vi "ge_Val2String_1Chan.vi"(0 "Value":u16, 1 "ColType":T1) -> (5 "String and Val":cluster{"String":string, "Value":u16})   [LabVIEW 2012]
uses:
  Custom Ctls Table/ge_ColType.ctl
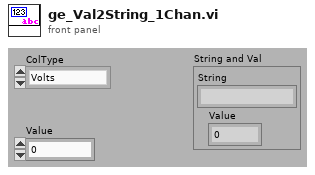
[diagram p1: front panel]
types:
  T1 = typedef "ge_ColType.ctl" = enum16{"Volts", "Amps", "Ohms", "TermCfg", "WireCfg", "Coup", "Slope", "Iex", "CalUnits", "ThrmUnits", "ThrmType", "CJCSrc", "BrdgType", "Strn Mode", "RTDType"}
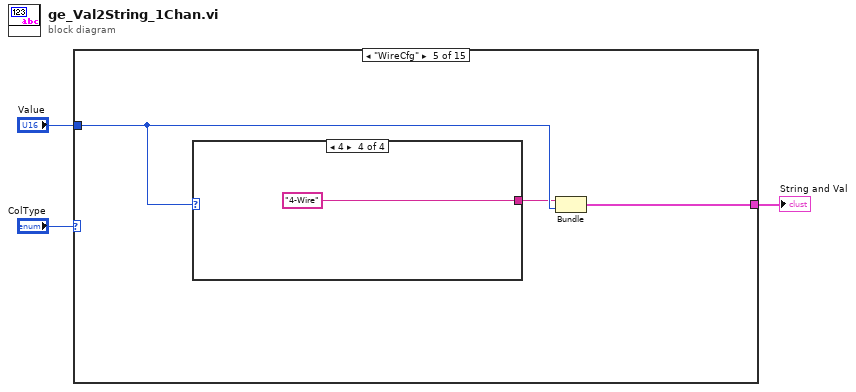
[diagram p0: block diagram]
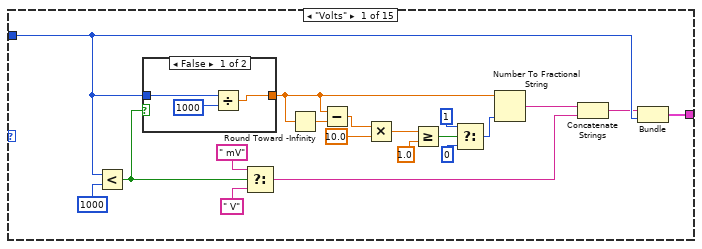
[diagram p2: hidden frame]
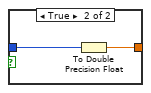
[diagram p3: hidden frame]
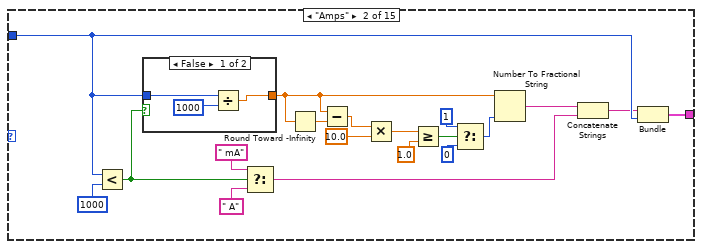
[diagram p4: hidden frame]
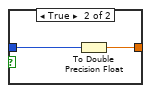
[diagram p5: hidden frame]
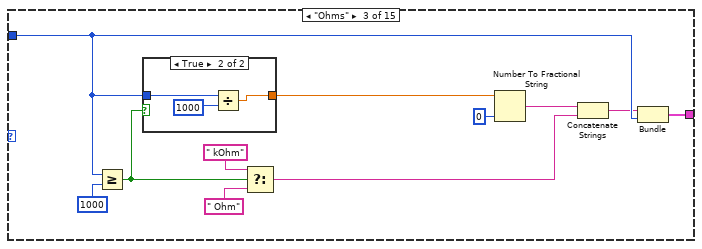
[diagram p6: hidden frame]
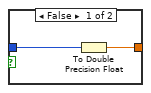
[diagram p7: hidden frame]
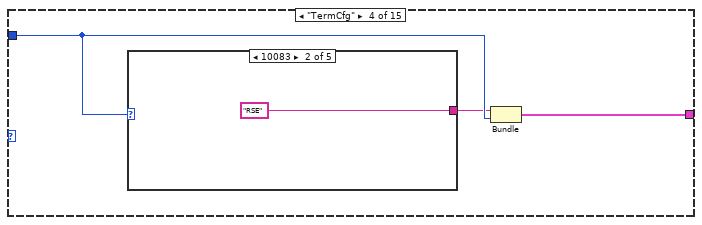
[diagram p8: hidden frame]
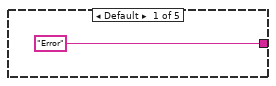
[diagram p9: hidden frame]
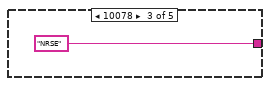
[diagram p10: hidden frame]
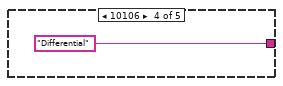
[diagram p11: hidden frame]
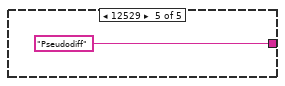
[diagram p12: hidden frame]
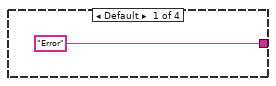
[diagram p13: hidden frame]
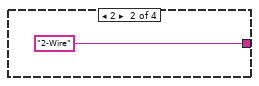
[diagram p14: hidden frame]
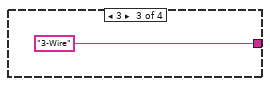
[diagram p15: hidden frame]
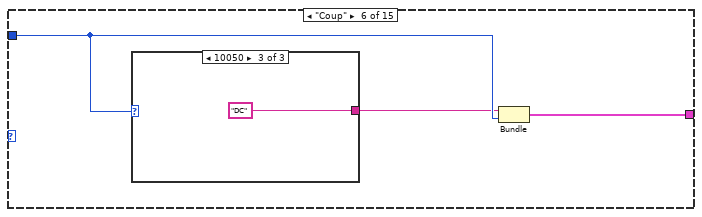
[diagram p16: hidden frame]
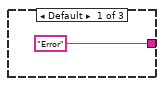
[diagram p17: hidden frame]
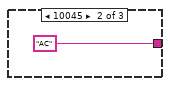
[diagram p18: hidden frame]
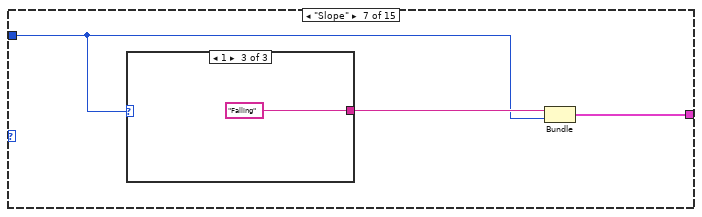
[diagram p19: hidden frame]
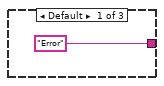
[diagram p20: hidden frame]
diagram:
  n1 = case shown="\"WireCfg\"" "ColType" {
    tunnel: "Value" -> [w22 w46 w62 w70 w78 w85 w89 w99 w101 w109 w117 w129 w135 w146 w152]
    tunnel: [w21 w45 w61 w69 w77 w84 w91 w98 w100 w108 w116 w128 w134 w145 w151] -> w1
    frame "Volts" {
      n2 = Less?(x=w22, y=1000) -> (x < y?=w14:bool)
      n3 = case shown="False" w14 {
        tunnel: w22 -> [w24 w27]
        tunnel: [w23 w26] -> w12
        frame False {
          n4 = Divide(x=w24, y=1000) -> (x/y=w23:dbl)
        }
        frame True {
          n5 = To Double Precision Float(number=w27) -> (double precision float=w26:dbl)
        }
      }
      n6 = Select(t=" mV" ("string"), s=w14, f=" V" ("string")) -> (s? t:f=w16:string)
      n7 = Round Toward -Infinity(1:w12) -> (0:w13:dbl)
      n8 = Subtract(x=w12, y=w13) -> (x-y=w11:dbl)
      n9 = Multiply(x=w11, y=10.0) -> (x*y=w9:dbl)
      n10 = Greater Or Equal?(x=w9, y=1.0) -> (x >= y?=w7:bool)
      n11 = Select(t=i16 1 ("precision (6)"), s=w7, f=i16 0 ("precision (6)")) -> (s? t:f=w4:i16)
      n12 = Number To Fractional String(number=w12, precision (6)=w4) -> (F-format string=w20:string)  [unwired: 2 in]
      n13 = Concatenate Strings(w20, w16) -> (w15:string)
      n14 = Bundle(w15, "Value"=w22) -> (w21:cluster{string, "Value":u16})  [unwired: 1 in]
    }
    frame "Amps" {
      n15 = Less?(x=w46, y=1000) -> (x < y?=w38:bool)
      n16 = case shown="False" w38 {
        tunnel: w46 -> [w48 w51]
        tunnel: [w47 w50] -> w36
        frame False {
          n17 = Divide(x=w48, y=1000) -> (x/y=w47:dbl)
        }
        frame True {
          n18 = To Double Precision Float(number=w51) -> (double precision float=w50:dbl)
        }
      }
      n19 = Select(t=" mA" ("string"), s=w38, f=" A" ("string")) -> (s? t:f=w40:string)
      n20 = Round Toward -Infinity(1:w36) -> (0:w37:dbl)
      n21 = Subtract(x=w36, y=w37) -> (x-y=w35:dbl)
      n22 = Multiply(x=w35, y=10.0) -> (x*y=w33:dbl)
      n23 = Greater Or Equal?(x=w33, y=1.0) -> (x >= y?=w31:bool)
      n24 = Select(t=i16 1 ("precision (6)"), s=w31, f=i16 0 ("precision (6)")) -> (s? t:f=w28:i16)
      n25 = Number To Fractional String(number=w36, precision (6)=w28) -> (F-format string=w44:string)  [unwired: 2 in]
      n26 = Concatenate Strings(w44, w40) -> (w39:string)
      n27 = Bundle(w39, "Value"=w46) -> (w45:cluster{string, "Value":u16})  [unwired: 1 in]
    }
    frame "Ohms" {
      n28 = Greater Or Equal?(x=w62, y=1000) -> (x >= y?=w54:bool)
      n29 = case shown="True" w54 {
        tunnel: w62 -> [w64 w66]
        tunnel: [w63 w65] -> w53
        frame False {
          n30 = To Double Precision Float(number=w64) -> (double precision float=w63:dbl)
        }
        frame True {
          n31 = Divide(x=w66, y=1000) -> (x/y=w65:dbl)
        }
      }
      n32 = Select(t=" kOhm" ("string"), s=w54, f=" Ohm" ("string")) -> (s? t:f=w56:string)
      n33 = Number To Fractional String(number=w53, precision (6)=i16 0) -> (F-format string=w60:string)  [unwired: 2 in]
      n34 = Concatenate Strings(w60, w56) -> (w55:string)
      n35 = Bundle(w55, "Value"=w62) -> (w61:cluster{string, "Value":u16})  [unwired: 1 in]
    }
    frame "TermCfg" {
      n36 = case shown="10083" w70 {
        tunnel: ["Error" "RSE" "NRSE" "Differential" "Pseudodiff"] -> w68
        frame Default {
        }
        frame 10083 {
        }
        frame 10078 {
        }
        frame 10106 {
        }
        frame 12529 {
        }
      }
      n37 = Bundle(w68, "Value"=w70) -> (w69:cluster{string, "Value":u16})  [unwired: 1 in]
    }
    frame "WireCfg" {
      n38 = case shown="4" w78 {
        tunnel: ["Error" "2-Wire" "3-Wire" "4-Wire"] -> w76
        frame Default {
        }
        frame 2 {
        }
        frame 3 {
        }
        frame 4 {
        }
      }
      n39 = Bundle(w76, "Value"=w78) -> (w77:cluster{string, "Value":u16})  [unwired: 1 in]
    }
    frame "Coup" {
      n40 = case shown="10050" w85 {
        tunnel: ["Error" "AC" "DC"] -> w83
        frame Default {
        }
        frame 10045 {
        }
        frame 10050 {
        }
      }
      n41 = Bundle(w83, "Value"=w85) -> (w84:cluster{string, "Value":u16})  [unwired: 1 in]
    }
    frame "Slope" {
      n42 = case shown="1" w89 {
        tunnel: ["Error" "Rising" "Falling"] -> w90
        frame Default {
        }
        frame 0 {
        }
        frame 1 {
        }
      }
      n43 = Bundle(w90, "Value"=w89) -> (w91:cluster{string, "Value":u16})  [unwired: 1 in]
    }
    frame "Iex" {
      n44 = Number To Decimal String(number=w99) -> (decimal integer string=w97:string)  [unwired: 1 in]
      n45 = Concatenate Strings(w97, " mA" ("string")) -> (w96:string)
      n46 = Bundle(w96, "Value"=w99) -> (w98:cluster{string, "Value":u16})  [unwired: 1 in]
    }
    frame "CalUnits" {
      n47 = case shown="2" w101 {
        tunnel: ["Error" "dB RMS" "EU Pk" "EU RMS"] -> w102
        frame Default {
        }
        frame 0 {
        }
        frame 1 {
        }
        frame 2 {
        }
      }
      n48 = Bundle(w102, "Value"=w101) -> (w100:cluster{string, "Value":u16})  [unwired: 1 in]
    }
    frame "ThrmUnits" {
      n49 = case shown="10145" w109 {
        tunnel: ["Error" "Deg C" "Deg F" "Kelvins" "Deg R"] -> w107
        frame Default {
        }
        frame 10143 {
        }
        frame 10144 {
        }
        frame 10325 {
        }
        frame 10145 {
        }
      }
      n50 = Bundle(w107, "Value"=w109) -> (w108:cluster{string, "Value":u16})  [unwired: 1 in]
    }
    frame "ThrmType" {
      n51 = case shown="10055" w117 {
        tunnel: ["Error" "J" "K" "N" "R" "S" "T" "B" "E"] -> w115
        frame Default {
        }
        frame 10072 {
        }
        frame 10073 {
        }
        frame 10077 {
        }
        frame 10082 {
        }
        frame 10085 {
        }
        frame 10086 {
        }
        frame 10047 {
        }
        frame 10055 {
        }
      }
      n52 = Bundle(w115, "Value"=w117) -> (w116:cluster{string, "Value":u16})  [unwired: 1 in]
    }
    frame "CJCSrc" {
      n53 = case shown="10116" w129 {
        tunnel: ["Error" "Built-In" "Const Val"] -> w127
        frame Default {
        }
        frame 10200 {
        }
        frame 10116 {
        }
      }
      n54 = Bundle(w127, "Value"=w129) -> (w128:cluster{string, "Value":u16})  [unwired: 1 in]
    }
    frame "BrdgType" {
      n55 = case shown="10185" w135 {
        tunnel: ["Error" "Full Bridge I" "Full Bridge II" "Full Bridge III" "Half Bridge I" "Half Bridge II" "Quarter Bridge I" "Quarter Bridge II"] -> w133
        frame Default {
        }
        frame 10183 {
        }
        frame 10184 {
        }
        frame 10185 {
        }
        frame 10188 {
        }
        frame 10189 {
        }
        frame 10271 {
        }
        frame 10272 {
        }
      }
      n56 = Bundle(w133, "Value"=w135) -> (w134:cluster{string, "Value":u16})  [unwired: 1 in]
    }
    frame "Strn Mode" {
      n57 = case shown="1" w146 {
        tunnel: ["Error" "High Res" "High Range"] -> w144
        frame Default {
        }
        frame 0 {
        }
        frame 1 {
        }
      }
      n58 = Bundle(w144, "Value"=w146) -> (w145:cluster{string, "Value":u16})  [unwired: 1 in]
    }
    frame "RTDType" {
      n59 = case shown="12483" w152 {
        tunnel: ["Error" "Pt3750" "Pt3851" "Pt3911" "Pt3916" "Pt3920" "Pt3928"] -> w150
        frame Default {
        }
        frame 12481 {
        }
        frame 10071 {
        }
        frame 12482 {
        }
        frame 10069 {
        }
        frame 10053 {
        }
        frame 12483 {
        }
      }
      n60 = Bundle(w150, "Value"=w152) -> (w151:cluster{string, "Value":u16})  [unwired: 1 in]
    }
  }
  "String and Val" <- w1
